vi "SignalGenerator_x410.vi"(10 "phase":fxp<+,64,64>, 11 "Reset":bool) -> (0 "data_valid":bool, 1 "Cos":fxp<+/-,18,1>, 2 "Sin":fxp<+/-,18,1>)   [LabVIEW 2025]
uses:
  <vilib>/rvi/IPIntegrationNode/IPINode_Typedef/niFpgaIPINodeSupportedFamilies.ctl
  <vilib>/rvi/FXPMathLib/FxpConvert/subVIs/nifxpmath_Convert_SimConfig.ctl
  <vilib>/fxp/LVFixedPointQuantizationPolicyTypeDef.ctl
  <vilib>/fxp/LVFixedPointOverflowPolicyTypeDef.ctl
  <vilib>/rvi/IPIntegrationNode/IPINode_Utilities/niFpgaIPINodeSimCore.vi
  <vilib>/rvi/FXPMathLib/FxpConvert/simVIs/DllFxpConvertTemp_sub.vi
  <vilib>/rvi/FXPMathLib/FxpInterpret/XNode/nifxpmath_Interpret.xnode
  <vilib>/rvi/XilinxIP/XIPIN_XNode/niFpgaXIPIN.xnode
  Xilinx/DDS_simulator/xsim.dir/DDS_Compiler_8AEA4D6678494B609559049F07B86E68/xsimk_8AEA4D6678494B609559049F07B86E68.dll
  <vilib>/rvi/IPIntegrationNode/IPINode_Xnode/niFpgaIPINode.xnode
  <vilib>/rvi/FXPMathLib/FxpConvert/XNode/nifxpmath_Convert.xnode
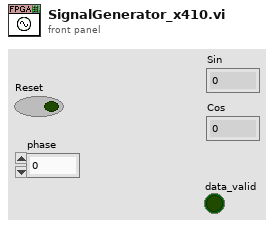
[diagram p1: front panel]
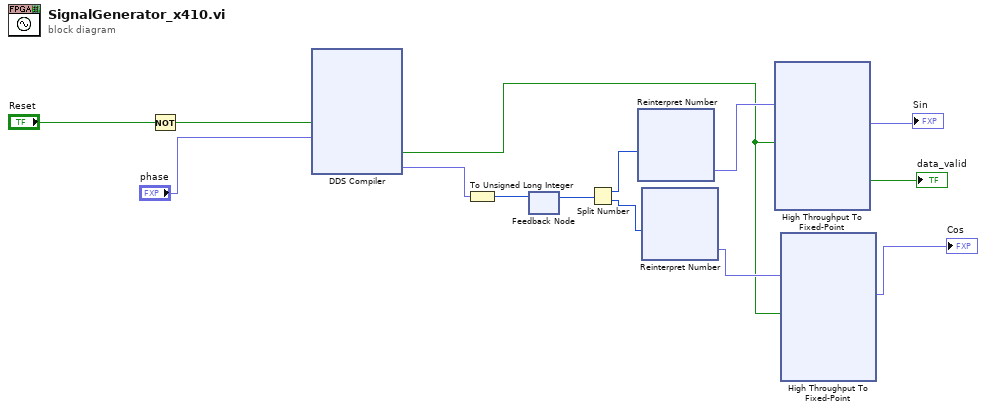
[diagram p0: block diagram]
diagram:
  n1 = Not(x="Reset") -> (.not. x?=w9:bool)
  n2 = xnode ("DDS Compiler")("aresetn"=w9, "s_axis_phase_tdata"="phase") -> ("m_axis_data_tvalid"=w1:bool, "m_axis_data_tdata"=w7:fxp<+,32,32>)  [unwired: 2 in]
  n3 = To Unsigned Long Integer(number=w7) -> (unsigned 32bit integer=w11:u32)
  n4 = feedback #1() -> (w10:u32)  [unwired: 1 in]
  n5 = feedback-in #1(w11) -> ()
  n6 = Split Number(x=w10) -> (hi(x)=w14:u16, lo(x)=w13:u16)
  n7 = xnode "Reinterpret Number"("x"=w14) -> ("y"=w6:fxp<+/-,16,0>)
  n8 = xnode "Reinterpret Number"("x"=w13) -> ("y"=w3:fxp<+/-,16,0>)
  n9 = xnode "High Throughput To Fixed-Point"("x"=w6, "input valid"=w1) -> ("y"=→"Sin":fxp<+/-,18,1>, "output valid"=→"data_valid":bool)  [unwired: 1 in, 1 out]
  n10 = xnode "High Throughput To Fixed-Point"("x"=w3, "input valid"=w1) -> ("y"=→"Cos":fxp<+/-,18,1>)  [unwired: 1 in, 2 out]
